vi "CaptureFromCamera (SubVI).vi"(8 "error in (no error)":errorcluster, 10 "Threshold Range":cluster{"Low value":dbl, "Upper value":dbl}, 11 "camera session in":T3) -> (0 "error out":errorcluster, 1 "Histogram Graph":T1 {"Incremental Value" format="%.2f"; "Starting Value" format="%.2f"}, 3 "image out":T2)   [LabVIEW 2016]
uses:
  <vilib>/userdefined/High Color/IMAQdx.ctl
  <vilib>/vision/Image Controls.llb/IMAQ Image.ctl
  <vilib>/vision/driver/NI_Vision_Acquisition_Software.lvlib
  <vilib>/vision/NI_Vision_Development_Module.lvlib
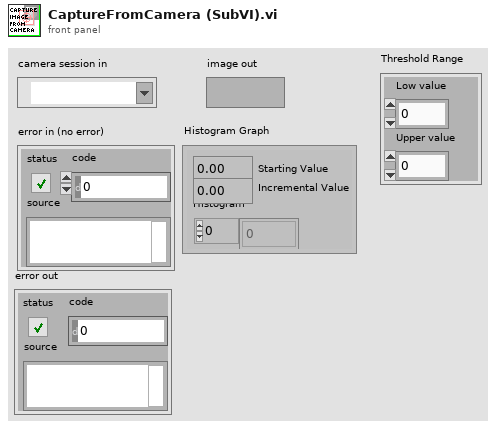
[diagram p1: front panel]
types:
  T1 = cluster{"Starting Value":sgl, "Incremental Value":sgl, "Histogram":u32[]}
  T2 = typedef "IMAQ Image.ctl" = refnum<image>
  T3 = typedef "IMAQdx.ctl" = refnum<k21>
  T4 = typedef "Image Type" = u32
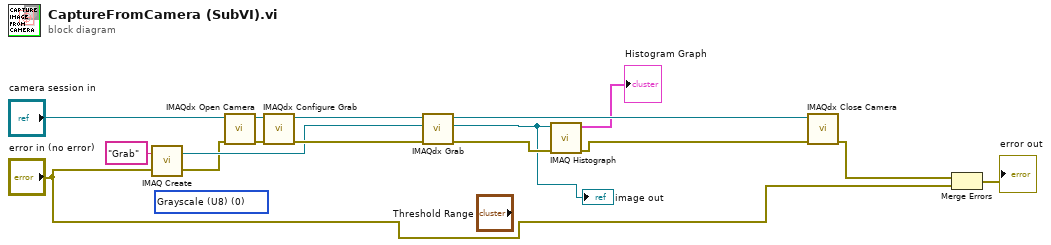
[diagram p0: block diagram]
diagram:
  (unwired) T4 0 items=["Grayscale (U8)", "Grayscale (I16)", "Grayscale (SGL)", "Complex (CSG)", "RGB (U32)", "HSL (U32)", "RGB (U64)", "Grayscale (U16)"] ("Image Type")
  n1 = call "IMAQ Create"("Image Name"="Grab", "error in (no error)"="error in (no error)") -> ("New Image"=w11:T2, "error out"=w5:errorcluster)  [unwired: 2 in, 1 out]
  n2 = call <vilib>:"IMAQdx Open Camera.vi"("error in"=w5, "Session In"="camera session in") -> ("error out"=w10:errorcluster, "Session Out"=w9:T3)  [unwired: 1 in, 7 out]
  n3 = call <vilib>:"IMAQdx Configure Grab.vi"("error in"=w10, "Session In"=w9) -> ("error out"=w13:errorcluster, "Session Out"=w12:T3)  [unwired: 8 out]
  n4 = call <vilib>:"IMAQdx Grab.vi"("error in"=w13, "Image In"=w11, "Session In"=w12) -> ("error out"=w3:errorcluster, "Image Out"=w1:T2, "Session Out"=w14:T3)  [unwired: 1 in, 5 out]
  "image out" <- w1
  n5 = call "IMAQ Histograph"("error in (no error)"=w3, "Image"=w1) -> ("error out"=w6:errorcluster, "Histogram Graph"=→"Histogram Graph":T1)  [unwired: 6 in, 2 out]
  n6 = call <vilib>:"IMAQdx Close Camera.vi"("error in"=w6, "Session In"=w14) -> ("error out"=w4:errorcluster)  [unwired: 9 out]
  n7 = Merge Errors(w4, "error in (no error)") -> (→"error out":errorcluster)
